vi "Do.vi"(8 "error in (no error)":errorcluster, 9 "Events":refnum<class "Events.lvclass">, 10 "Message Loop Data in":T1, 11 "IInternalRequest in":refnum<class "IResultHandler.lvclass">) -> (0 "error out":errorcluster, 2 "Message Loop Data out":T1, 3 "IInternalRequest out":refnum<class "IResultHandler.lvclass">)   [LabVIEW 2020, in "wamplv.lvlib" / "IResultHandler.lvclass"]
uses:
  IResultHandler.lvclass
  Call/ICallRequest/ICallRequest.lvclass
  WAMP Client/Private/TypeDef/Publish Requests Map.ctl
  wamplv.lvlib
  WAMP Client/Private/TypeDef/Endpoint Data.ctl
  WAMP Client/Private/TypeDef/CALL Request Map.ctl
  WAMP Client/Private/TypeDef/SUBSCRIBE Requests Map.ctl
  WAMP Client/Private/TypeDef/Subscriptions Map.ctl
  WAMP Client/Private/TypeDef/Unsubscribe Requests Map.ctl
  WAMP Client/Private/TypeDef/Unregister requests map.ctl
  WAMP Client/Private/TypeDef/Message Loop Data.ctl
  Events/EventsParent/Events.lvclass
  Subscribe/ISubscribe/ISubscribe.lvclass
  Publish/IPublish/IPublish.lvclass
  Message loop classes/Subscription details/SubscriptionDetailsParent/SubscriptionDetailsParent.lvclass
  Unsubscribe/IUnsubscribe/IUnsubscribe.lvclass
  Register/IRegister/IRegister.lvclass
  Unregister/IUnregister/IUnregister.lvclass
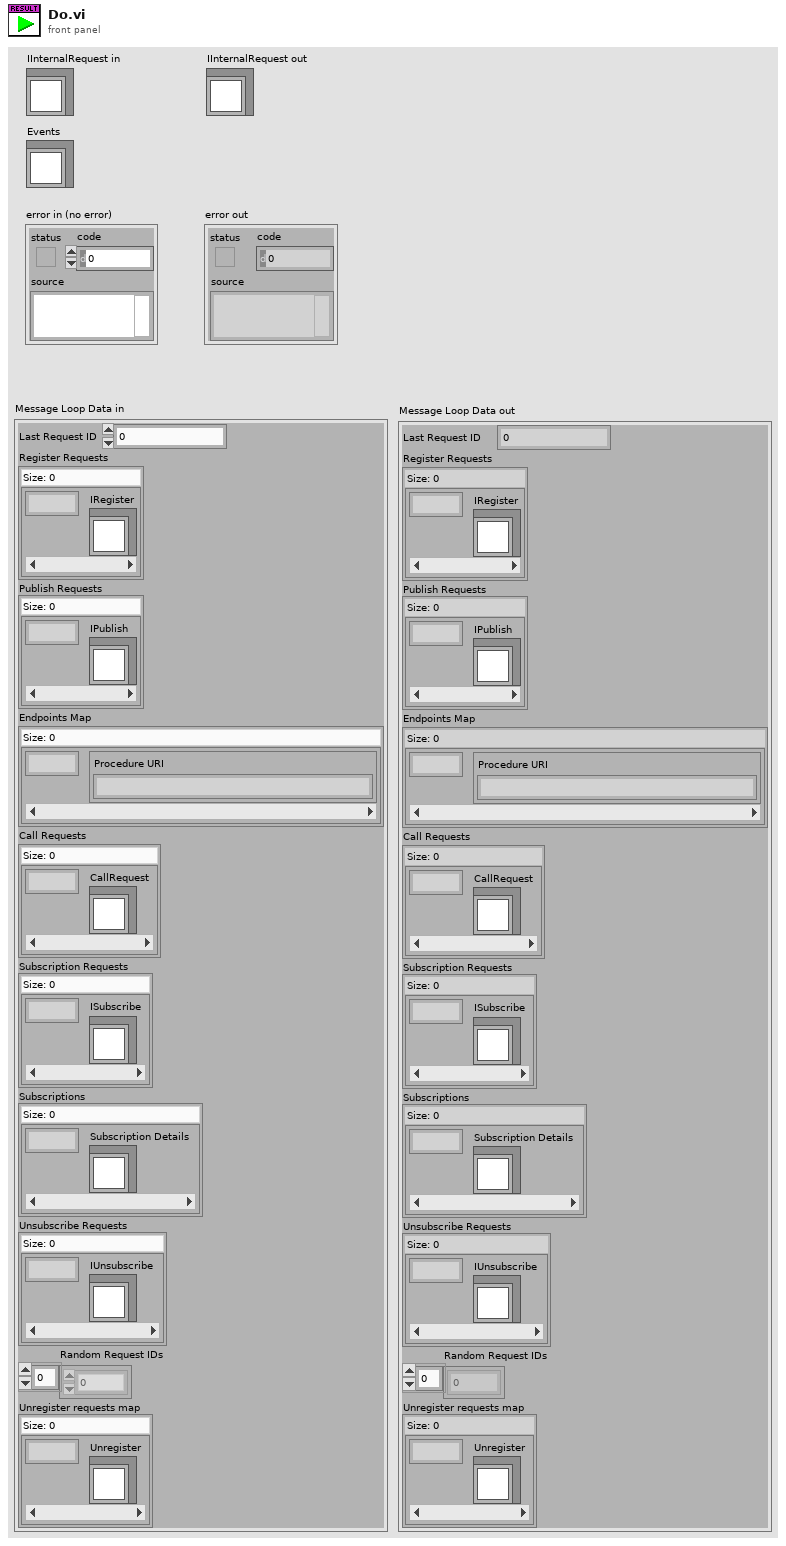
[diagram p1: front panel]
types:
  T1 = typedef "wamplv.lvlib/Message Loop Data.ctl" = cluster{"Last Request ID":u64, "Register Requests":map{u64, refnum<class "IRegister.lvclass">}, "Publish Requests":T2, "Endpoints Map":map{u64, T3}, "Call Requests":T4, "Subscription Requests":T5, "Subscriptions":T6, "Unsubscribe Requests":T7, "Random Request IDs":u64[], "Unregister requests map":T8}
  T2 = typedef "wamplv.lvlib/Publish Requests Map.ctl" = map{u64, refnum<class "IPublish.lvclass">}
  T3 = typedef "wamplv.lvlib/Endpoint Data.ctl" = cluster{"Procedure URI":string}
  T4 = typedef "wamplv.lvlib/CALL Request Map.ctl" = map{u64, refnum<class "ICallRequest.lvclass">}
  T5 = typedef "wamplv.lvlib/SUBSCRIBE Requests Map.ctl" = map{u64, refnum<class "ISubscribe.lvclass">}
  T6 = typedef "wamplv.lvlib/Subscriptions Map.ctl" = map{u64, refnum<class "SubscriptionDetailsParent.lvclass">}
  T7 = typedef "wamplv.lvlib/Unsubscribe Requests Map.ctl" = map{u64, refnum<class "IUnsubscribe.lvclass">}
  T8 = typedef "wamplv.lvlib/Unregister requests map.ctl" = map{u64, refnum<class "IUnregister.lvclass">}
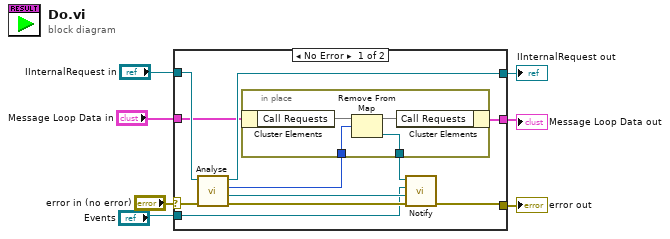
[diagram p0: block diagram]
diagram:
  n1 = case shown="No Error" "error in (no error)" {
    selector: "error in (no error)" -> [w16 w25]
    tunnel: "IInternalRequest in" -> [w18 w23]
    tunnel: [w17 w23] -> w6
    tunnel: "Message Loop Data in" -> [w14 w24]
    tunnel: [w13 w24] -> w3
    tunnel: "Events" -> [w9 _]
    tunnel: [w8 w25] -> w1
    frame No Error {
      n2 = call-dynamic "Analyse.vi"("error in (no error)"=w16, "IResultHandler in"=w18) -> ("error out"=w11:errorcluster, "ICallResult"=w10:refnum<class "ICallResult.lvclass">, "Request ID"=w15:u64, "IResultHandler out"=w17:refnum<class "IResultHandler.lvclass">)  [unwired: 6 in]
      n3 = in-place "In Place Element Structure" {
        in-place-border: w15 -> [w22]
        in-place-border: [w21] -> w12
        n4 = in-place-cluster #1(w14) -> ("Call Requests"=w20:T4)
        n5 = Remove From Map(10:w22, 11:w20) -> (1:w21:refnum<class "ICallRequest.lvclass">, 3:w19:T4)  [unwired: 1 out]
        n6 = in-place-cluster #1("Call Requests"=w19) -> (w13:T1)
      }
      n7 = call-dynamic "Notify.vi"("error in (no error)"=w11, "ICallResult"=w10, "Events"=w9, "ICallRequest in"=w12) -> ("error out"=w8:errorcluster)  [unwired: 6 in, 1 out]
    }
    frame Error {
    }
  }
  "error out" <- w1
  "IInternalRequest out" <- w6
  "Message Loop Data out" <- w3
